vi "hardware_serial.vi"(6 "timeout (25000ms)":i32=25000, 8 "error in (no error)":errorcluster, 11 "daemon reference in":refnum<k5>) -> (0 "error out":errorcluster, 1 "hardware_serial":string, 2 "response":string, 3 "daemon reference out":refnum<k5>, 5 "command out":string="random")   [LabVIEW 2017]
doc: "<b>Command: </b>\"template\"\n\n<b>Description: </b> This command does something.\n\n<b>Parameters: </b> None\n____________________________________________\nDIPC 692 Daemon API 10.0.0.1\nSam Tee - Dyson Technology Ltd\nCopyright (c) 2024, Dyson Technology Ltd"
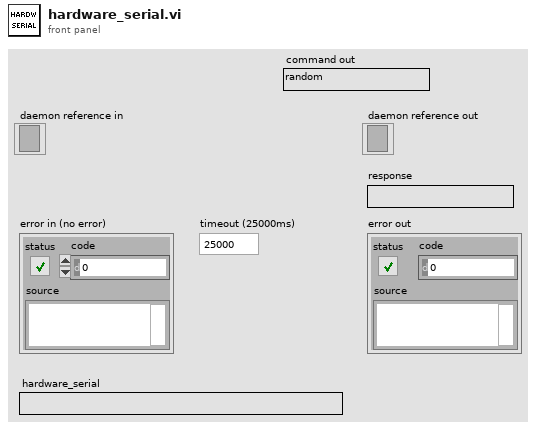
[diagram p1: front panel]
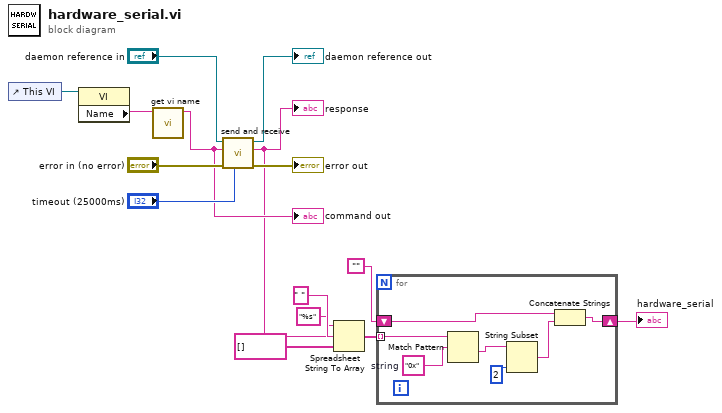
[diagram p0: block diagram]
diagram:
  n1 = control-ref of="This VI"() -> (w10:refnum<vi>)
  n2 = property class="VI"(reference=w10) -> ("Name"=w9:string)  [unwired: 1 in, 2 out]
  n3 = call "get vi name.vi"("library.lvlib:name.vi"=w9) -> ("vi name"=w8:string)  [unwired: 10 in]
  "command out" <- w8
  n4 = call "send and receive.vi"("timeout (25000ms)"="timeout (25000ms)", "error in (no error)"="error in (no error)", "command"=w8, "daemon reference in"="daemon reference in") -> ("error out"=→"error out":errorcluster, "response"=w2:string, "daemon reference out"=→"daemon reference out":refnum<k5>)  [unwired: 5 in]
  "response" <- w2
  n5 = Spreadsheet String To Array(delimiter (Tab)=" ", format string="%s", spreadsheet string=w2, array type (2D Dbl)=string[] []) -> (array=w3:string[])
  n6 = for {
    tunnel: w3 -> [w22] mode=indexing
    shift-right: [w19] -> w1
    shift-left: "" -> [w20]
    w21 = "0x"  # string
    n7 = Match Pattern(string=w22, regular expression=w21) -> (after substring=w17:string)  [unwired: 1 in, 3 out]
    n8 = String Subset(string=w17, length (rest)=2 ("y")) -> (substring=w16:string)  [unwired: 1 in]
    n9 = Concatenate Strings(w20, w16) -> (w19:string)
  }
  "hardware_serial" <- w1
